vi "OLD_Dashboard_Main_Fixed_1280_768.vi"() -> ()   [LabVIEW 2025]
uses:
  frobotics-2025RobotCode/2025ReefBot/Intake/IntakeStates.ctl
  frobotics-2025RobotCode/2025ReefBot/NewAuto/NewAutoStepTypeEnum.ctl
  <vilib>/event_ctls.llb/eventvkey.ctl
  frobotics-2025RobotCode/Dashboard-Testing/Dash_Globals.vi
  <vilib>/Rock Robotics/Network Tables/NT Read Boolean.vi
  <vilib>/Rock Robotics/Network Tables/NT Write Boolean.vi
  <vilib>/Rock Robotics/WPI/Dashboard/WPI_DashboardLogging Global.vi
  <vilib>/Rock Robotics/WPI/ThirdParty/JAS_Junk/TrajLib/Trajectory_Library.lvlib
panel:
  in  "Camera Settings Right":T1={"Frame Rate"=30, "Compression"=30, "Size"=1, "DB Camera Config"=FALSE} {"Frame Rate" scale=1.0..30.0; "Compression" scale=100.0..-1.0; "Size" items=["640x480", "320x240", "160x120"]}
  in  "Camera Name Right":string(combo)="No Camera Selection"
  out "Camera Perf":string
  in  "Camera Settings":T1={"Frame Rate"=30, "Compression"=30, "Size"=1, "DB Camera Config"=FALSE} {"Frame Rate" scale=1.0..30.0; "Compression" scale=100.0..-1.0; "Size" items=["640x480", "320x240", "160x120"]}
  in  "TCP":refnum<k5>
  in  "Rec Mode":enum32{"Stop", "Record", "Playback"}(radio)
  out "Robot IP":string
  out "Image Message":string="Timeout in Camera Communications"
  in  "Dashboard Tab":T2(tab)
  out "Human Fast Turn":bool
  out "H Traj Orient Deg":dbl format="%11.2f"
  out "H Traj Y Ft":dbl format="%11.2f"
  out "H Traj X Ft":dbl format="%11.2f"
  out "Human Slow Mode":bool
  out "Human Field Orient":bool
  out "A String":string
  out "P3":dbl format="%11.2f"
  out "Function":T3
  out "A Step":i64 format="%11.0f"
  out "P2":dbl format="%11.2f"
  out "P1":dbl format="%11.2f"
  out "TO":dbl format="%11.2f"
  out "Vision Targets Found":bool
  out "Climb Position":dbl format="%15.2f"
  out "Climb Status":string
  out "Fully Pulled":bool
  out "Fully Reached":bool
  out "Intake State":T4
  out "Have Algae":bool
  out "Have Coral":bool
  out "W PV":dbl(slide) scale=-90.0..90.0
  out "W SP":dbl(slide) scale=-90.0..90.0
  out "W Hi Clamp":bool
  out "W Lo Clamp":bool
  out "W On Tgt":bool
  out "W Motor":dbl format="%11.2f"
  out "W Pos Deg":dbl format="%12.1f"
  out "W Dmd Deg":dbl format="%12.1f"
  out "I PV":dbl(slide) scale=0.0..26.0
  out "I SP":dbl(slide) scale=0.0..26.0
  out "I Lo Clamp":bool
  out "I Lo Lim":bool
  out "I Hi Lim":bool
  out "I On Tgt":bool
  out "I Motor":dbl format="%11.2f"
  out "I Pos In":dbl format="%12.1f"
  out "I Dmd In":dbl format="%12.1f"
  in  "Select Auto":string(combo)="Select Autonomous ..."
  out "NT Connection":bool
  out "Mode":T5(ring)=enum."Auto Disabled"
  out "Right Camera Perf":cluster{"Bandwidth (Mbps)":dbl, "FPS":dbl}
  out "Selected Auto":string
  out "O PV":dbl(slide) scale=0.0..52.0
  out "O SP":dbl(slide) scale=0.0..52.0
  out "O Lo Lim":bool
  out "O Hi Lim":bool
  out "O On Tgt":bool
  out "O Motor":dbl format="%11.2f"
  out "O Pos In":dbl format="%12.1f"
  out "O Dmd In":dbl format="%12.1f"
  out "Camera Image Right":T6(plugin-control)
  out "AlgSensOffDlyFB":dbl
  in  "AlgSensOffDly":dbl
  out "AlgSensOnDlyFB":dbl
  in  "AlgSensOnDly":dbl
  out "AlgHoldMtrFB":dbl
  in  "AlgHoldMtr":dbl
  in  "Alg Update":bool
  out "AlgIntakeMtrFB":dbl
  in  "AlgIntakeMtr":dbl
  out "Max Amb FB":dbl
  in  "Max Amb":dbl
  out "I Orient Deg FB":dbl
  in  "Init Orient Deg":dbl
  out "InitYPosFt FB":dbl
  in  "InitYPos Ft":dbl
  in  "Vision Update":bool
  out "InitXPos Ft FB":dbl
  in  "InitXPos Ft":dbl
  out "RL Enable FB":bool
  in  "RL Enable":bool
  out "Y Acc M/S2 FB":dbl
  in  "Y Acc M/S2":dbl
  in  "RL Update":bool
  out "X Acc M/S2 FB":dbl
  in  "X Acc M/S2":dbl
  in  "RA Update":bool
  out "R Starting Angle FB":dbl
  in  "R Starting Angle":dbl
  in  "LQR":bool
  in  "Filter":bool
  out "Wrist Chart":T7(graph)
  out "Kp Calc":dbl
  out "Kg FB":dbl
  in  "Kg":dbl
  out "Kd FB":dbl format="%#_7g"
  in  "Kd":dbl format="%#_7g"
  out "Output Max FB":dbl
  in  "Output Max":dbl
  out "Output DB FB":dbl
  in  "Output DB":dbl
  out "Error DB FB":dbl
  in  "Error DB":dbl
  in  "WR Tune Update":bool
  out "Error Thres FB":dbl
  in  "Error Thres":dbl
  out "Filt FB":bool
  out "LQR FB":bool
  in  "Test Slider":dbl(slide) scale=0.0..100.0 scale format="%#_3g"
  in  "On/Off":bool caption="Solenoid"
  in  "Test Name":u16(ring) items=["Select the test to run..."]
  in  "Test Tree":string(tree)
  in  "Motor":cluster{"Value":dbl, "Enable":bool} {"Value" scale=-1.0..1.0 scale format="%#_3g"}
  out "Progress":T8 {"Test Progress" scale=0.0..100.0}
  in  "Rev/Fwd":cluster{"Forward":bool, "Reverse":bool}
  in  "Test Ring":u16(ring) items=["Monochrome", "Color"]
  in  "CheckList":i32(listbox)
  out "Tree":string(tree)
  out "Camera Image":T6(plugin-control)
  out "Background":bool
  in  "Camera Name":string(combo)="No Camera Selection"
  # "HW"
  # "HW"
  # "Human"
  # "Auto"
  # "VISION"
  # "CLIMB"
  # "INTAKE"
  # "WRIST"
  # "INNER ELEV"
  # "OUTER ELEV"
  # "Intake Algae Tuning"
  # "Vision Tuning"
  # "Drive Rate Limiting"
  # "Initial Robot Angle"
  # "Wrist Tuning"
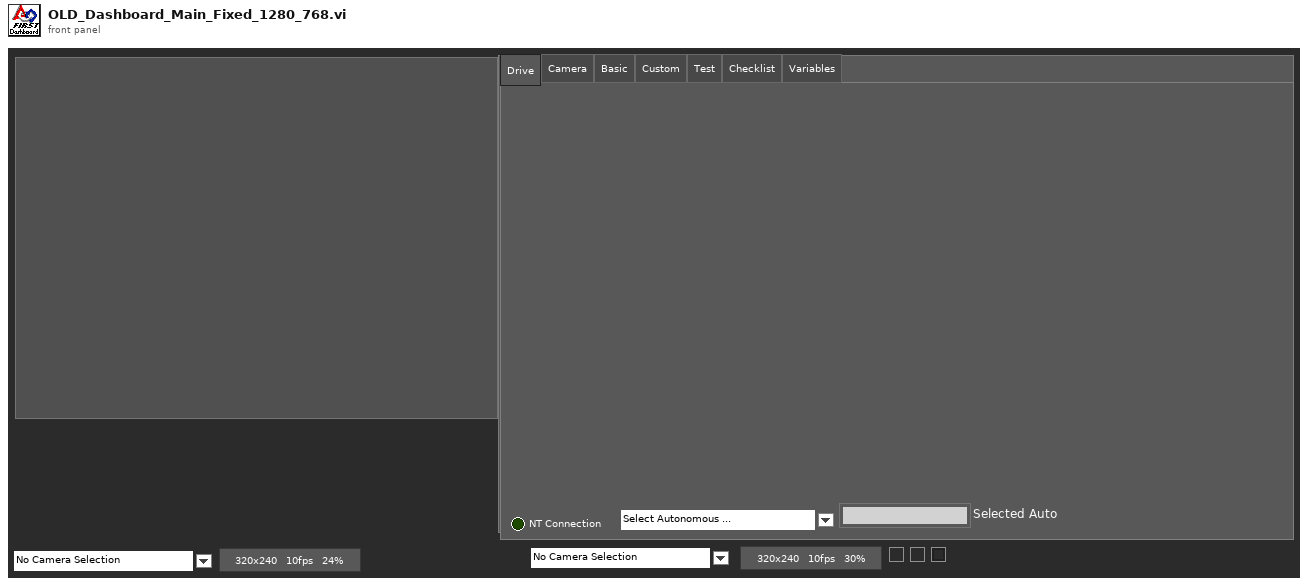
[diagram p1: front panel]
types:
  T1 = cluster{"Frame Rate":i32, "Compression":i32, "Size":u16, "DB Camera Config":bool}
  T2 = enum32{"Drive", "Camera", "Basic", "Custom", "Test", "Checklist", "Variables"}
  T3 = typedef "NewAutoStepTypeEnum.ctl" = enum16{"DriveStraight", "DriveTurn", "FollowAbsoluteTrajectory", "FollowRelativeTrajectory", "AutoWait", "ElevToRest", "ElevToFloor", "ElevToSource", "ElevToL1", "ElevToL2", "ElevToL3", "ElevToL4", "ElevToAlgae1", "ElevToAlgae2", "ElevToBarge", "ElevCancel", "IntakeCoral", "IntakeAlgae", "IntakeDepositCoral", "IntakeDepositAlgae", "IntakeCancel", "ElevRestWait", "ElevFloorWait", "ElevSourceWait", "ElevL1Wait", "ElevL2Wait", "ElevAlgae1Wait", "ElevL3Wait", "ElevAlgae2Wait", "ElevL4Wait", "ElevBargeWait", "IntakeWait", "FollowAbsTrajWithTimedCmd", "FollowRelTrajWithTimedCmd"}
  T4 = typedef "IntakeStates.ctl" = enum16{"Start", "WaitForCommand", "IntakeCoral", "IntakeAlgae", "WaitForCoral", "WaitForAlgae", "DepositCoral", "DepositAlgae", "DepositCoralTimer", "DepositAlgaeTimer"}
  T5 = enum8{"Tele-Op Disabled", "Tele-Op Enabled", "Auto Disabled", "Auto Enabled", "Test Disabled", "Test Enabled", "Disconnected", "No Code", "E-Stop"}
  T6 = typedef "IMAQ Image.ctl" = refnum<image>
  T7 = cluster{"WristSetpointDeg":dbl, "WristPosDeg":dbl, "WristMotorDmd":dbl, "WristGravityCompMotorDmd":dbl}
  T8 = cluster{"Test Progress":u8, "Test Progress Text":string}
  T9 = cluster{"Save Path":path, "Interval (s)":dbl, "Keep":i32}
  T10 = typedef "Image Type" = u32
  T11 = enum32{"Drive", "Camera", "Basic", "Custom", "Test", "Commands", "Checklist", "Variables"}
  T12 = cluster{"Error Strings":string, "Disable Counts":cluster{u16, u16}, "Rail Faults":cluster{u16, u16, u16}, "Robot IP":string, "DB Mode":u8, "Event Info":cluster{"Name":string, "Type":u8, "Number":u16, "Replay":u8}}
  T13 = cluster{"Storage":cluster{"Disk Free":u64, "RAM Block":u32, "RAM free":u32}, "CPU Utilization":cluster{"CPU % ISR":sgl, "CPU % Time Crit":sgl, "CPU % Timed Str":sgl, "CPU % High":sgl, "CPU % Above":sgl, "CPU % Normal":sgl, "CPU % Low":sgl}, "CAN":cluster{"% Bus Utilization":sgl, "Bus Off Cnt":u32, "TX_FIFO Full Cnt":u32, "Receive Error Cnt":u8, "Transmit Error Cnt":u8}, "HID":cluster{"HID Outputs":u32, "Rumble Low":u16, "Rumble High":u16}[]}
  T14 = cluster{"Status bits":cluster{"Test Mode":bool, "Autonomous":bool, "Enabled":bool, "Code Start":bool, "Brownout":bool, "Reserved 2":bool, "Reserved 3":bool, "E-Stop":bool}, "Code Trace":cluster{"Disabled":bool, "TeleOp":bool, "Auto":bool, "Test":bool}, "Controller Type":enum16{"unknown", "cRIO", "roboRio"}, "Code?":enum16{"unknown", "noCode", "code"}, "Battery V":dbl}
  T15 = cluster{"Control Bits":cluster{"TestMode":bool, "Autonomous":bool, "Enabled":bool, "FMS Present":bool, bool, bool, bool, "E-Stop":bool}, "Team Station ":u8, "Countdown":sgl, "Joystick Values":cluster{"Axes":dbl[], "Buttons":bool[], "POVs":i16[]}[]}
  T16 = cluster{"Camera Image":refnum<vi>, "Dashboard Tab":refnum<vi>, "Background":refnum<vi>, "Rec Mode":refnum<vi>, "Test Slider":refnum<vi>, "On/Off ":refnum<vi>, "Test Ring":refnum<vi>, "Rev/Fwd":refnum<vi>, "Test Name":refnum<vi>, "Motor":refnum<vi>, "Progress":refnum<vi>, "CheckList":refnum<vi>, "Tree":refnum<vi>, "Test Tree":refnum<vi>, "Camera Settings":refnum<vi>, "Camera Name":refnum<vi>, "Camera Perf":refnum<vi>, "Camera Settings Right":refnum<vi>, "Camera Name Right":refnum<vi>, "Camera Image Right":refnum<vi>}
  T17 = cluster{"Global Rectangle":i32[], "Contours":cluster{"Contour Type":u32, "ROI Type":u32, "Points":i32[]}[]}
  T18 = cluster{"Camera Name":string, string, "Saved DB Images Info":cluster{"Save Path":path, "Interval (s)":dbl, "Keep":i32}}
  T19 = cluster{"Camera Name Right":string, string, "Saved DB Images Info":cluster{"Save Path":path, "Interval (s)":dbl, "Keep":i32}}
  T20 = cluster{"Operation":enum16{"Update", "Clear"}, "Color Box":u32}[]
  T21 = typedef "eventvkey.ctl" = enum16{"ASCII", "Enter", "Return", "Shift", "Ctrl", "Alt", "Cmd", "Opt", "Caps", "NumLock", "Clear", "Break", "Up", "Down", "Left", "Right", "Insert", "Delete", "Home", "End", "PageUp", "PageDown", "Escape", "Help", "Pause", "ScrollLock", "F1", "F2", "F3", "F4", "F5", "F6", "F7", "F8", "F9", "F10", "F11", "F12", "F13", "F14", "F15", "F16", "F17", "F18", "F19", "F20", "F21", "F22", "F23", "F24", "Play", "VolumeUp", "VolumeDown", "Mute", "Two Byte Char"}
  T22 = cluster{"Image Size":bool, "Image Type":bool, "Pixel Value":bool, "ROI Information":bool, "Zoom Factor":bool}
  T23 = cluster{"Operation":enum16{"Update", "Clear"}, "Color Box":u32}
  T24 = cluster{"Shift":bool, "Ctrl":bool, "Alt":bool, "Cmd":bool, "Opt":bool}
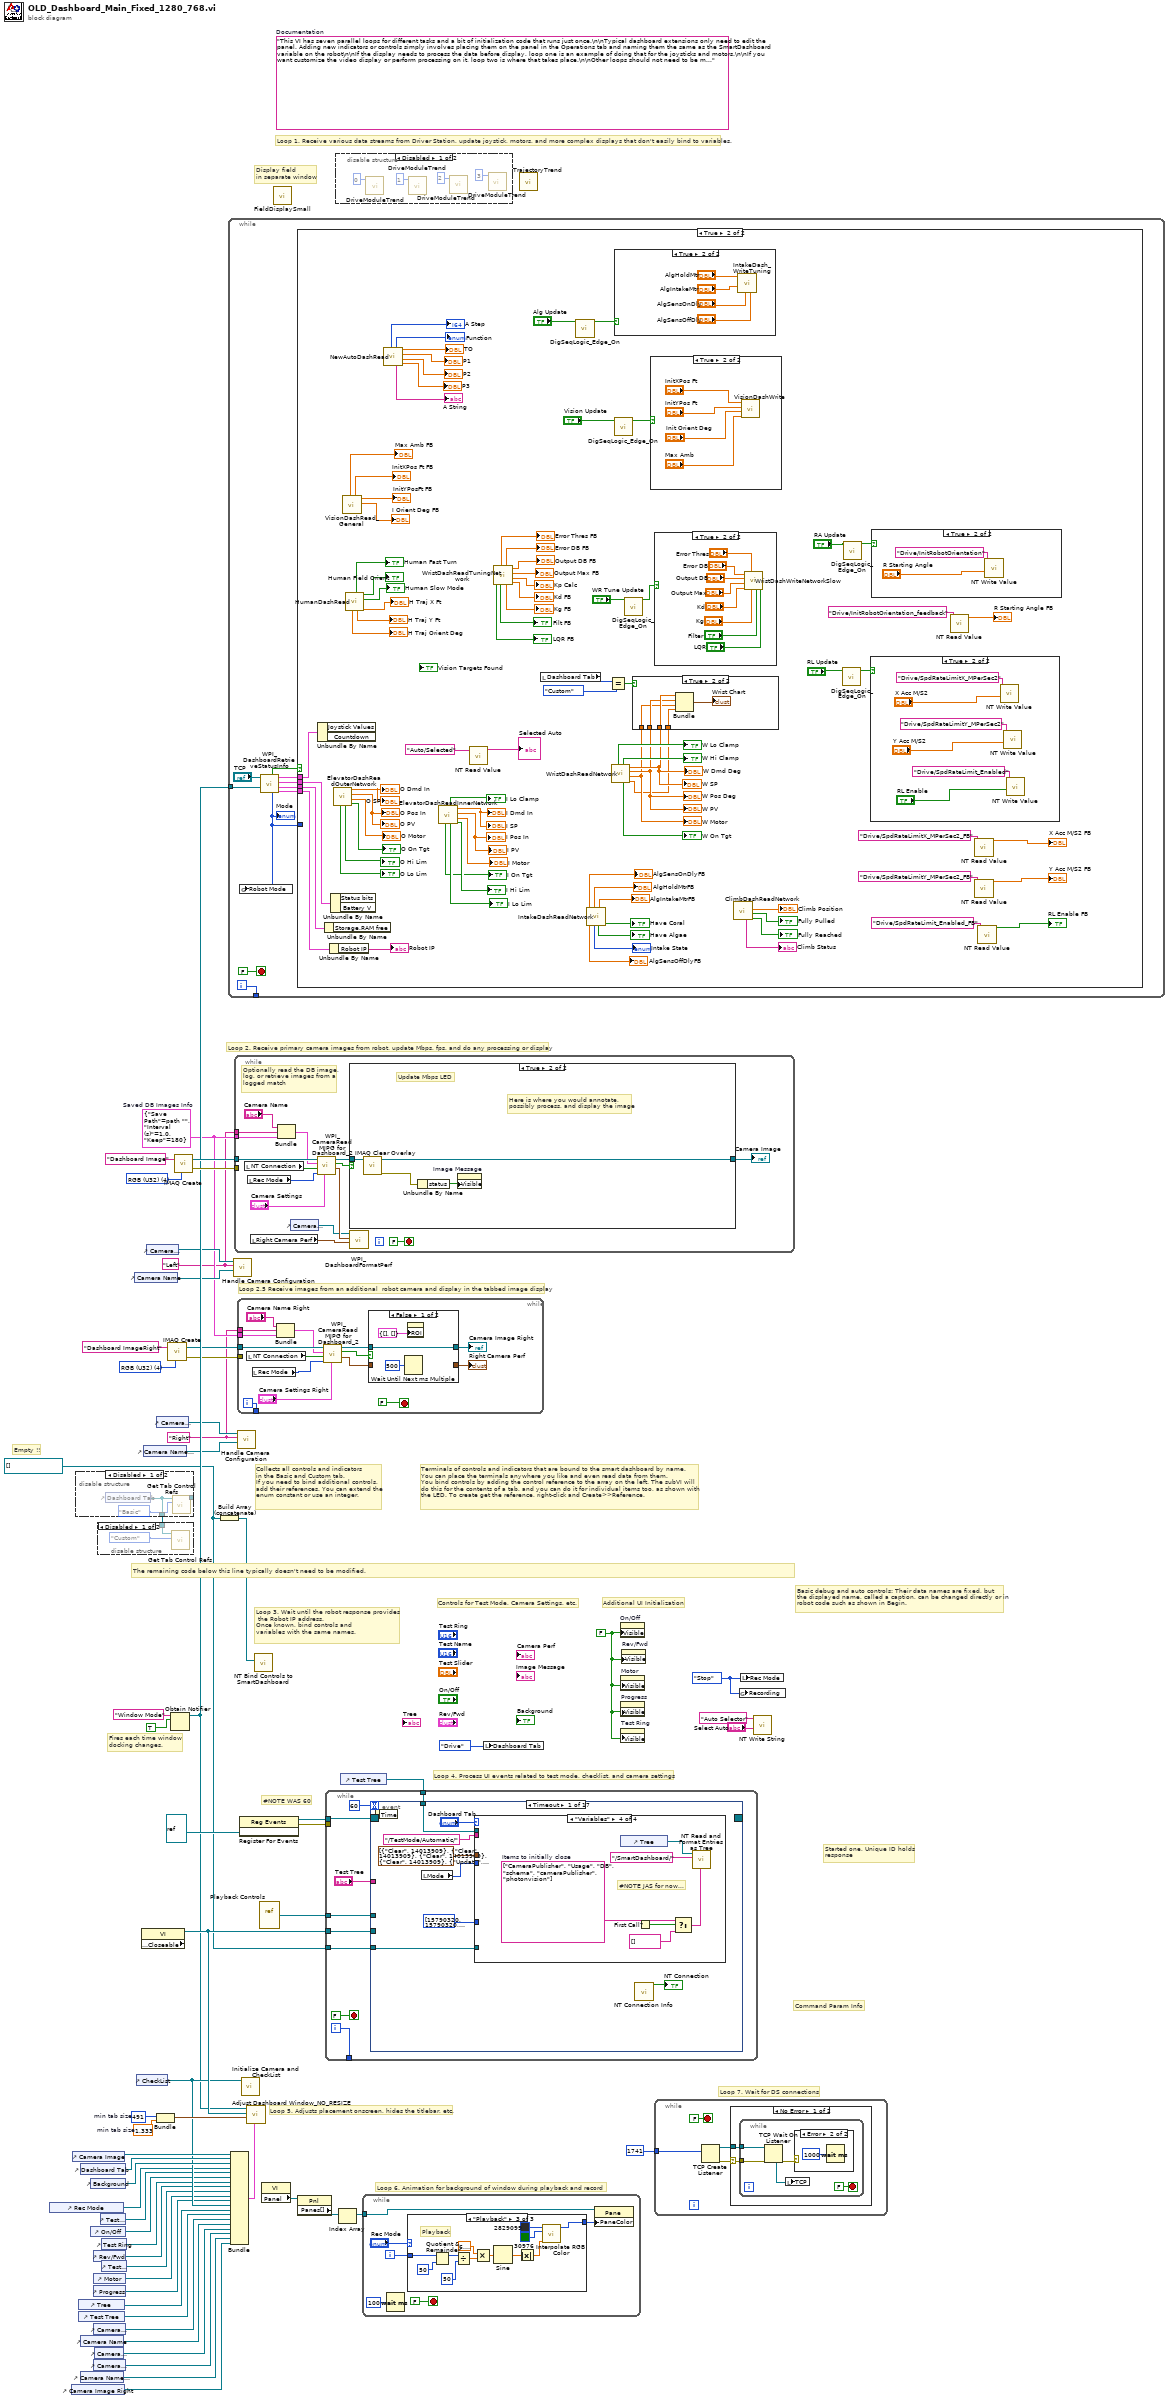
[diagram p0: block diagram]
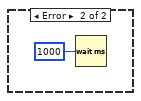
[diagram p7: hidden frame]
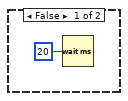
[diagram p8: hidden frame]
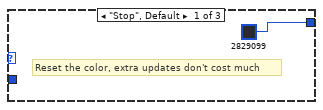
[diagram p15: hidden frame]
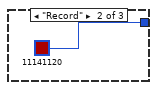
[diagram p16: hidden frame]
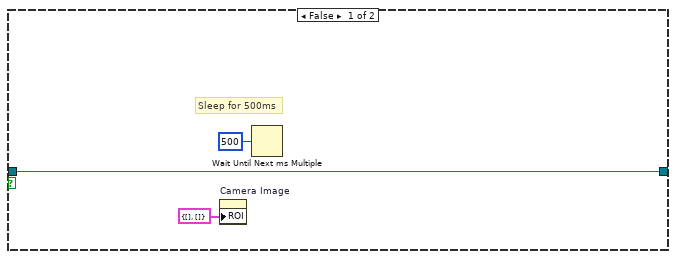
[diagram p17: hidden frame]
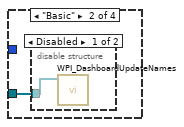
[diagram p19: hidden frame]
diagram:
  w1 = refnum<vi>[] [] ("ControlsOnPage")
  w4 = T9 {"Save Path"=path "", "Interval (s)"=1.0, "Keep"=180}  # Saved DB Images Info
  w3 = "Right"
  w2 = "Left"
  w12 = T10 4 items=["Grayscale (U8)", "Grayscale (I16)", "Grayscale (SGL)", "Complex (CSG)", "RGB (U32)", "HSL (U32)", "RGB (U64)"] ("Image Type")
  w40 = 491  # min tab size
  w39 = 1.333  # min tab size
  w46 = enum32{"Stop", "Record", "Playback"}."Stop" ("Rec Mode")
  w24 = FALSE ("Visible")
  (unwired) "This VI has seven parallel loops for different tasks and a bit of initialization code that runs just once.\n\nTypical dashboard extensions only need to edit the panel. Adding new indicators or controls simply involves placing them on the panel in the Operations tab and naming them the same as the SmartDashboard variable on the robot\n\nIf the display needs to process the data before display, loop one is an example of doing that for the joysticks and motors.\n\nIf you want customize the video display or perform processing on it, loop two is where that takes place.\n\nOther loops should not need to be modified. They are pretty standard, and document the task they perform."  # Documentation
  w60 = T10 4 items=["Grayscale (U8)", "Grayscale (I16)", "Grayscale (SGL)", "Complex (CSG)", "RGB (U32)", "HSL (U32)", "RGB (U64)"] ("Image Type")
  # "#NOTE WAS 60"
  # "Empty !!"
  # "Display field\nin separate window"
  # "Loop 2.5 Receive images from an additional  robot camera and display in the tabbed image display"
  # "Command Param Info"
  # "Started one, Unique ID holds\nresponse"
  # "Loop 7. Wait for DS connections"
  # "Basic debug and auto controls: Their data names are fixed, but\nthe displayed name, called a caption, can be changed directly or in\nrobot code such as shown in Begin."
  # "Controls for Test Mode, Camera Settings, etc."
  # "Additional UI Initialization"
  # "Loop 6. Animation for background of window during playback and record"
  # "Fires each time window\ndocking changes."
  # "Collects all controls and indicators\nin the Basic and Custom tab.\nIf you need to bind additional controls,\nadd their references. You can extend the\nenum constant or use an integer."
  # "The remaining code below this line typically doesn't need to be modified."
  # "Loop 4. Process UI events related to test mode, checklist, and camera settings"
  # "Terminals of controls and indicators that are bound to the smart dashboard by name.\nYou can place the terminals anywhere you like and even read data from them.\nYou bind controls by adding the control reference to the array on the left. The subVI will\ndo this for the contents of a tab, and you can do it for individual items too, as shown with\nthe LED. To create get the reference, right-click and Create>>Reference."
  # "Loop 3. Wait until the robot response provides\n the Robot IP address.\nOnce known, bind controls and\nvariables with the same names."
  # "Loop 5. Adjusts placement onscreen, hides the titlebar, etc."
  # "Loop 1. Receive various data streams from Driver Station, update joystick, motors, and more complex displays that don't easily bind to variables."
  # "Loop 2. Receive primary camera images from robot, update Mbps, fps, and do any processing or display"
  n1 = control-ref of="Rec Mode"() -> (w30:refnum<vi>)
  n2 = control-ref of="Camera Image Right"() -> (w5:refnum<vi>)
  n3 = control-ref of="Camera Image"() -> (w42:refnum<vi>)
  n4 = disable-structure shown="Disabled" {
    disable-tunnel: [w63 _] -> w44
    disable-tunnel: [w62 _] -> _
    frame Disabled {
      n5 = control-ref of="Dashboard Tab"() -> (w63:refnum<vi>)
      n6 = call <vilib>:"Get Tab Control Refs.vi"("Page Index"=T11."Basic" ("Dashboard Tab"), "TabControl in"=w63) -> ("ControlsOnPage"=w62:refnum<vi>[])  [unwired: 9 in]
    }
    frame Enabled {
    }
  }
  n7 = control-ref of="Tree"() -> (w34:refnum<vi>)
  n8 = control-ref of="Test Tree"() -> (w33:refnum<vi>)
  n9 = control-ref of="Dashboard Tab"() -> (w41:refnum<vi>)
  n10 = control-ref of="Camera Name"() -> (w17:refnum<vi>)
  n11 = control-ref of="Camera Name Right"() -> (w6:refnum<vi>)
  n12 = control-ref of="Background"() -> (w37:refnum<vi>)
  n13 = control-ref of="On/Off"() -> (w28:refnum<vi>)
  n14 = control-ref of="Progress"() -> (w25:refnum<vi>)
  n15 = control-ref of="Camera Settings"() -> (w18:refnum<vi>)
  n16 = control-ref of="Camera Settings Right"() -> (w7:refnum<vi>)
  n17 = control-ref of="Rev/Fwd"() -> (w26:refnum<vi>)
  n18 = control-ref of="Motor"() -> (w31:refnum<vi>)
  n19 = control-ref of="Camera Perf"() -> (w16:refnum<vi>)
  n20 = disable-structure shown="Disabled" {
    disable-tunnel: w44 -> [w65 _]
    frame Disabled {
      n21 = call <vilib>:"Get Tab Control Refs.vi"("Page Index"=T11."Custom" ("Dashboard Tab"), "TabControl in"=w65) -> ()  [unwired: 9 in, 1 out]
    }
    frame Enabled {
    }
  }
  n22 = control-ref of="Test Slider"() -> (w29:refnum<vi>)
  n23 = control-ref of="Test Ring"() -> (w27:refnum<vi>)
  n24 = control-ref of="Test Name"() -> (w32:refnum<vi>)
  n25 = control-ref of="Camera Name"() -> (w19:refnum<vi>)
  n26 = control-ref of="CheckList"() -> (w35:refnum<vi>)
  n27 = property class="VI" props=["Front Panel.Closeable"]() -> (reference out=w45:refnum<vi>)  [unwired: 2 in, 2 out]
  n28 = control-ref of="Camera Name Right"() -> (w8:refnum<vi>)
  n29 = control-ref of="Camera Settings"() -> (w20:refnum<vi>)
  n30 = control-ref of="Camera Settings Right"() -> (w9:refnum<vi>)
  n31 = Bundle("min tab size"=w40, "min tab size"=w39) -> (w38:cluster{"min tab size":i32, "min tab size":dbl})  [unwired: 1 in]
  n32 = call "IMAQ Create"("Image Name"="Dashboard ImageRight", "Image Type"=w12) -> ("New Image"=w11:T6, "error out"=w10:errorcluster)  [unwired: 2 in, 1 out]
  n33 = Obtain Notifier(name (unnamed)="Window Mode", notification data type=TRUE) -> (notifier out=w23:refnum<notifier>)  [unwired: 2 in, 2 out]
  n34 = call "IMAQ Create"("Image Name"="Dashboard Image", "Image Type"=w60) -> ("New Image"=w58:T6, "error out"=w57:errorcluster)  [unwired: 2 in, 1 out]
  n35 = Build Array (concatenate)(w1) -> (w43:refnum<vi>[])
  n36 = while {
    tunnel: [w74] -> _
    tunnel: w23 -> [w67]
    i -> [w74]
    stop <- FALSE stop-if-true
    n37 = call <vilib>:"WPI_DashboardRetrieveStatusInfo.vi"("Window Mode Notifier"=w67, "TCP Cnx"="TCP") -> ("Power and Errors"=w69:T12, "Robot Metrics"=w72:T13, "Status Info"=w73:T14, "Control Info"=w70:T15, "Robot Mode"=w66:T5, "Process?"=w71:bool)  [unwired: 4 in]
    "Mode" <- w66
    n38 = global write "Dash_Globals.vi" "Robot Mode"(w66) -> ()
    n39 = case shown="True" w71 {
      tunnel: w73 -> [_ w161]
      tunnel: w72 -> [_ w160]
      tunnel: w70 -> [_ w159]
      tunnel: w69 -> [_ w158]
      tunnel: w66 -> [_ _]
      frame False {
        n40 = Wait (ms)(milliseconds to wait=u32 20) -> ()  [unwired: 1 out]
      }
      frame True {
        n41 = Unbundle By Name(w159) -> ()  [unwired: 2 out]
        n42 = Unbundle By Name(w160) -> ()  [unwired: 1 out]
        n43 = Unbundle By Name(w158) -> ("Robot IP"=→"Robot IP":string)
        n44 = Unbundle By Name(w161) -> ()  [unwired: 2 out]
        n45 = call "ElevatorDashReadOuterNetwork.vi"() -> ("OuterOnTarget"=→"O On Tgt":bool, "OuterMotorOutput"=→"O Motor":dbl, "OuterPositionHeight"=→"O PV" →"O Pos In":dbl, "OuterPosDemandHeight"=→"O SP" →"O Dmd In":dbl, "OuterHighLimitSwitch"=→"O Hi Lim":bool, "OuterLowLimitSwitch"=→"O Lo Lim":bool)  [unwired: 6 in]
        n46 = call "VisionDashRead_General.vi"() -> ("InitOrientDeg"=→"I Orient Deg FB":dbl, "InitYFt"=→"InitYPosFt FB":dbl, "InitXFt"=→"InitXPos Ft FB":dbl, "MaxAmbiguity"=→"Max Amb FB":dbl)  [unwired: 4 in, 4 out]
        n47 = call "HumanDashRead.vi"() -> ("TrajDestX_Ft"=→"H Traj X Ft":dbl, "SlowMode"=→"Human Slow Mode":bool, "FieldOriented"=→"Human Field Orient":bool, "TrajDestY_Ft"=→"H Traj Y Ft":dbl, "FastMode"=→"Human Fast Turn":bool, "TrajDestAng_Deg"=→"H Traj Orient Deg":dbl)  [unwired: 5 in, 1 out]
        n48 = call "NewAutoDashRead.vi"() -> ("P3"=→"P3":dbl, "P2"=→"P2":dbl, "P1"=→"P1":dbl, "Timeout"=→"TO":dbl, "StepString"=→"A String":string, "StepType"=→"Function":T3, "StepIndex"=→"A Step":i64)  [unwired: 5 in]
        n49 = call "ElevatorDashReadInnerNetwork.vi"() -> ("Stage3HighLimitSwitch"=→"I Hi Lim":bool, "Stage3MotorOutput"=→"I Motor":dbl, "Stage3PositionHeight"=→"I Pos In" →"I PV":dbl, "Stage3PosDemandHeight"=→"I Dmd In" →"I SP":dbl, "Stage3LowLimitSwitch"=→"I Lo Lim":bool, "Stage3LowWristClampActive"=→"I Lo Clamp":bool, "Stage3OnTarget"=→"I On Tgt":bool)  [unwired: 5 in]
        n50 = call-poly <vilib>:"NT Read Value.vi"("name"="Auto/Selected") -> ("value"=→"Selected Auto":string)  [unwired: 8 in, 2 out]
        n51 = call "WristDashReadTuningNetwork.vi"() -> ("Tune_Kd"=→"Kd FB":dbl, "Tune_Kp"=→"Kp Calc":dbl, "Tune_OutMax"=→"Output Max FB":dbl, "Tune_OutDb"=→"Output DB FB":dbl, "Tune_Kg"=→"Kg FB":dbl, "Tune_ErrDb"=→"Error DB FB":dbl, "FilterDerivative"=→"Filt FB":bool, "Tune_ErrThres"=→"Error Thres FB":dbl, "UseLQR"=→"LQR FB":bool)  [unwired: 3 in]
        n52 = local read "Dashboard Tab"() -> (w109:T2)
        n53 = call <vilib>:"DigSeqLogic_Edge_On.vi"("Input"="Alg Update") -> ("On Edge"=w82:bool)  [unwired: 10 in]
        n54 = call "IntakeDashReadNetwork.vi"() -> ("HaveCoralSensor"=→"Have Coral":bool, "HaveAlgaeSensor"=→"Have Algae":bool, "AlgaeIntakeMtr"=→"AlgIntakeMtrFB":dbl, "CurrentState"=→"Intake State":T4, "AlgaeHoldMtr"=→"AlgHoldMtrFB":dbl, "AlgaeSensorOffDelaySec"=→"AlgSensOffDlyFB":dbl, "AlgaeSensorOnDelaySec"=→"AlgSensOnDlyFB":dbl)  [unwired: 2 in, 3 out]
        n55 = Equal?(x=w109, y=T2."Custom") -> (x = y?=w110:bool)
        n56 = call "WristDashReadNetwork.vi"() -> ("WristGravityCompMotorDmd"=w102:dbl, "WristMotorDmd"=w105:dbl, "WristPosDeg"=w106:dbl, "WristSetpointDeg"=w107:dbl, "WristAtSetpoint"=→"W On Tgt":bool, "WristProtectHighClampActive"=→"W Hi Clamp":bool, "WristProtectLowClampActive"=→"W Lo Clamp":bool)  [unwired: 5 in]
        "W Dmd Deg" <- w107
        "W Pos Deg" <- w106
        "W Motor" <- w105
        "W SP" <- w107
        "W PV" <- w106
        n57 = case shown="True" w82 {
          frame False {
          }
          frame True {
            n58 = call "IntakeDash_WriteTuning.vi"("AlgaeSensorOffDelaySec"="AlgSensOffDly", "AlgaeSensorOnDelaySec"="AlgSensOnDly", "AlgaeIntakeMtr"="AlgIntakeMtr", "AlgaeHoldMtr"="AlgHoldMtr") -> ()  [unwired: 8 in]
          }
        }
        n59 = call <vilib>:"DigSeqLogic_Edge_On.vi"("Input"="Vision Update") -> ("On Edge"=w100:bool)  [unwired: 10 in]
        n60 = call <vilib>:"DigSeqLogic_Edge_On.vi"("Input"="WR Tune Update") -> ("On Edge"=w112:bool)  [unwired: 10 in]
        n61 = case shown="True" w110 {
          tunnel: w107 -> [_ w173]
          tunnel: w106 -> [_ w172]
          tunnel: w105 -> [_ w171]
          tunnel: w102 -> [_ w170]
          frame False {
          }
          frame True {
            n62 = Bundle("WristSetpointDeg"=w173, "WristPosDeg"=w172, "WristMotorDmd"=w171, "WristGravityCompMotorDmd"=w170) -> (→"Wrist Chart":T7)  [unwired: 1 in]
          }
        }
        n63 = case shown="True" w100 {
          frame False {
          }
          frame True {
            n64 = call "VisionDashWrite.vi"("MaxAmbiguity"="Max Amb", "InitialOrientationDeg"="Init Orient Deg", "InitialYPositionFt"="InitYPos Ft", "InitialXPositionFt"="InitXPos Ft") -> ()  [unwired: 8 in]
          }
        }
        n65 = case shown="True" w112 {
          frame False {
          }
          frame True {
            n66 = call "WristDashWriteNetworkSlow.vi"("UseLQR"="LQR", "FilterDerivative"="Filter", "Tune_Kg"="Kg", "Tune_ErrThres"="Error Thres", "Tune_Kd"="Kd", "Tune_OutMax"="Output Max", "Tune_OutDb"="Output DB", "Tune_ErrDb"="Error DB") -> ()  [unwired: 4 in]
          }
        }
        n67 = call "ClimbDashReadNetwork.vi"() -> ("ReachLimit"=→"Fully Reached":bool, "PullLimit"=→"Fully Pulled":bool, "SensorPosition"=→"Climb Position":dbl, "ClimbStatus"=→"Climb Status":string)  [unwired: 7 in, 1 out]
        n68 = call <vilib>:"DigSeqLogic_Edge_On.vi"("Input"="RL Update") -> ("On Edge"=w126:bool)  [unwired: 10 in]
        n69 = call <vilib>:"DigSeqLogic_Edge_On.vi"("Input"="RA Update") -> ("On Edge"=w128:bool)  [unwired: 10 in]
        n70 = case shown="True" w126 {
          frame False {
          }
          frame True {
            n71 = call-poly <vilib>:"NT Write Value.vi"("value"="X Acc M/S2", "name"="Drive/SpdRateLimitX_MPerSec2") -> ()  [unwired: 9 in, 1 out]
            n72 = call-poly <vilib>:"NT Write Value.vi"("value"="Y Acc M/S2", "name"="Drive/SpdRateLimitY_MPerSec2") -> ()  [unwired: 9 in, 1 out]
            n73 = call-poly <vilib>:"NT Write Value.vi"("value"="RL Enable", "name"="Drive/SpdRateLimit_Enabled") -> ()  [unwired: 9 in, 1 out]
          }
        }
        n74 = case shown="True" w128 {
          frame False {
          }
          frame True {
            n75 = call-poly <vilib>:"NT Write Value.vi"("value"="R Starting Angle", "name"="Drive/InitRobotOrientation") -> ()  [unwired: 9 in, 1 out]
          }
        }
        n76 = call-poly <vilib>:"NT Read Value.vi"("name"="Drive/InitRobotOrientation_feedback") -> ("value"=→"R Starting Angle FB":dbl)  [unwired: 8 in, 2 out]
        n77 = call-poly <vilib>:"NT Read Value.vi"("name"="Drive/SpdRateLimitX_MPerSec2_FB") -> ("value"=→"X Acc M/S2 FB":dbl)  [unwired: 8 in, 2 out]
        n78 = call-poly <vilib>:"NT Read Value.vi"("name"="Drive/SpdRateLimitY_MPerSec2_FB") -> ("value"=→"Y Acc M/S2 FB":dbl)  [unwired: 8 in, 2 out]
        n79 = call-poly <vilib>:"NT Read Value.vi"("name"="Drive/SpdRateLimit_Enabled_FB") -> ("value"=→"RL Enable FB":bool)  [unwired: 8 in, 2 out]
      }
    }
  }
  n80 = Bundle("Camera Image"=w42, "Dashboard Tab"=w41, "Background"=w37, "Rec Mode"=w30, "Test Slider"=w29, "On/Off"=w28, "Test Ring"=w27, "Rev/Fwd"=w26, "Test Name"=w32, "Motor"=w31, "Progress"=w25, "CheckList"=w35, "Tree"=w34, "Test Tree"=w33, "Camera Settings"=w18, "Camera Name"=w17, "Camera Perf"=w16, "Camera Settings Right"=w7, "Camera Name Right"=w6, "Camera Image Right"=w5) -> (w36:T16)  [unwired: 1 in]
  n81 = call "Handle Camera Configuration.vi"("CameraNameRef"=w19, "Display Name"=w2, "ClusterRef"=w20) -> ()  [unwired: 9 in]
  n82 = while {
    tunnel: w58 -> [w204]
    tunnel: w57 -> [_]
    tunnel: w4 -> [w197]
    tunnel: w2 -> [w194]
    stop <- FALSE stop-if-true
    # "Optionally read the DB image,\nlog, or retrieve images from a\nlogged match"
    n83 = local read "NT Connection"() -> (w198:bool)
    n84 = local read "Rec Mode"() -> (w201:enum32{"Stop", "Record", "Playback"})
    n85 = local read "Right Camera Perf"() -> (w192:cluster{"Bandwidth (Mbps)":dbl, "FPS":dbl})
    n86 = Bundle("Camera Name"="Camera Name", w194, "Saved DB Images Info"=w197) -> (w196:T18)  [unwired: 1 in]
    n87 = control-ref of="Camera Perf"() -> (w191:refnum<vi>)
    n88 = call <vilib>:"WPI_CameraRead MJPG for Dashboard_2.vi"("Camera Settings"="Camera Settings", "Rec Mode"=w201, "NT Connection"=w198, "Capture Info"=w196, "Image in"=w204) -> ("perf info"=w193:cluster{"Bandwidth (Mbps)":dbl, "fps":dbl}, "Active"=w202:bool, "Image\\ out"=w203:T6)  [unwired: 4 in]
    n89 = case shown="True" w202 {
      tunnel: w203 -> [w207 w210]
      tunnel: [w207 w209] -> w199
      frame False {
        # "Sleep for 500ms"
        n90 = property on="Camera Image" class="ImageControl"("ROI"=T17 {"Global Rectangle"=[], "Contours"=[]}) -> ()  [unwired: 2 in, 2 out]
        n91 = Wait Until Next ms Multiple(millisecond multiple=u32 500) -> ()  [unwired: 1 out]
      }
      frame True {
        # "Here is where you would annotate,\npossibly process, and display the image"
        # "Update Mbps LED"
        n92 = call "IMAQ Clear Overlay"("Image"=w210) -> ("error out"=w211:errorcluster, "Image Out"=w209:T6)  [unwired: 2 in, 7 out]
        n93 = Unbundle By Name(w211) -> ("status"=w212:bool)
        n94 = property on="Image Message" class="Str"("Visible"=w212) -> ()  [unwired: 2 in, 2 out]
      }
    }
    "Camera Image" <- w199
    n95 = call <vilib>:"WPI_DashboardFormatPerf.vi"("Right Camera Perf"=w192, "Performance"=w193, "String in"=w191) -> ()  [unwired: 9 in]
  }
  n96 = call "Handle Camera Configuration.vi"("CameraNameRef"=w8, "Display Name"=w3, "ClusterRef"=w9) -> ()  [unwired: 9 in]
  n97 = while {
    tunnel: w11 -> [w227]
    tunnel: w10 -> [_]
    tunnel: [w222] -> _
    tunnel: w4 -> [w218]
    tunnel: w3 -> [w215]
    i -> [w222]
    stop <- FALSE stop-if-true
    n98 = local read "NT Connection"() -> (w219:bool)
    n99 = local read "Rec Mode"() -> (w226:enum32{"Stop", "Record", "Playback"})
    n100 = Bundle("Camera Name Right"="Camera Name Right", w215, "Saved DB Images Info"=w218) -> (w217:T19)  [unwired: 1 in]
    n101 = call <vilib>:"WPI_CameraRead MJPG for Dashboard_2.vi"("Camera Settings"="Camera Settings Right", "Rec Mode"=w226, "NT Connection"=w219, "Capture Info"=w217, "Image in"=w227) -> ("perf info"=w213:cluster{"Bandwidth (Mbps)":dbl, "fps":dbl}, "Active"=w221:bool, "Image\\ out"=w224:T6)  [unwired: 4 in]
    n102 = case shown="False" w221 {
      tunnel: w224 -> [w229 w232]
      tunnel: [w229 w232] -> w220
      tunnel: [_ w231] -> w214
      tunnel: w213 -> [_ w231]
      frame False {
        n103 = Wait Until Next ms Multiple(millisecond multiple=u32 500) -> ()  [unwired: 1 out]
        n104 = property on="Camera Image Right" class="ImageControl"("ROI"=T17 {"Global Rectangle"=[], "Contours"=[]}) -> ()  [unwired: 2 in, 2 out]
      }
      frame True {
      }
    }
    "Camera Image Right" <- w220
    "Right Camera Perf" <- w214
  }
  n105 = register-events(refnum<vi> refnum) -> (reference out=w49:refnum<event-registration>, error out=w48:errorcluster)  [unwired: 2 in]
  n106 = call "Initialize Camera and CheckList.vi"("ListBox in"=w35) -> ()  [unwired: 11 in]
  n107 = call "Adjust Dashboard Window_NO_RESIZE.vi"("Sizing Refnums"=w36, "Size Constraints"=w38, "VI"=w45, "WIn Mode"=w23) -> ()  [unwired: 8 in]
  n108 = call <vilib>:"NT Bind Controls to SmartDashboard.vi"("Bound Control Refs"=w43) -> ()  [unwired: 11 in]
  n109 = vi-ref "Playback Controls.vi"() -> (w50:refnum<vi>)
  n110 = property class="VI"() -> ("Panel"=w52:refnum<vi>)  [unwired: 2 in, 2 out]
  n111 = call "FieldDisplaySmall.vi"() -> ()  [unwired: 1 in]
  n112 = property class="Pnl"(reference=w52) -> ("Panes[]"=w53:refnum<vi>[])  [unwired: 1 in, 2 out]
  n113 = disable-structure shown="Disabled" {
    frame Disabled {
      n114 = call "DriveModuleTrend.vi"("Module"=0) -> ()  [unwired: 11 in]
      n115 = call "DriveModuleTrend.vi"("Module"=1) -> ()  [unwired: 11 in]
      n116 = call "DriveModuleTrend.vi"("Module"=2) -> ()  [unwired: 11 in]
      n117 = call "DriveModuleTrend.vi"("Module"=3) -> ()  [unwired: 11 in]
    }
    frame Enabled {
    }
  }
  n118 = Index Array(array=w53) -> (element=w51:refnum<vi>)  [unwired: 1 in]
  n119 = control-ref of="Test Tree"() -> (w54:refnum<vi>)
  n120 = while {
    tunnel: [w242] -> _
    tunnel: w54 -> [w241]
    tunnel: w50 -> [w240]
    tunnel: w49 -> [w239]
    tunnel: w48 -> [_]
    tunnel: w45 -> [w238]
    tunnel: w1 -> [w237]
    i -> [w242]
    stop <- FALSE stop-if-true
    n121 = event shown="[0] Timeout" {
      selector: w239 -> [_ _ _ _ _ _ _ _ _ _ _ _ _ _ _ _ _]
      dyn-events: [_ _ _ _ _ _ _ _ _ _ _ _ _ w449 _ _ _] -> _
      timeout: u32 60 ("milliseconds to wait") -> [_ _ _ _ _ _ _ _ _ _ _ _ _ _ _ _ _]
      tunnel: w241 -> [w252 _ _ _ _ _ _ _ _ _ _ _ _ _ _ _ _]
      tunnel: "Test Tree" -> [_ _ _ _ _ _ _ _ w422 w429 w430 w433 w440 _ _ _ _]
      tunnel: w240 -> [_ _ _ _ _ _ _ _ _ _ _ _ _ w451 _ w466 _]
      tunnel: w238 -> [_ _ _ _ _ _ _ _ _ _ _ _ _ w447 _ _ _]
      tunnel: w237 -> [w247 _ _ _ _ _ _ _ _ _ _ _ _ _ _ _ _]
      event Timeout {
        n122 = event-data() -> ()  [unwired: 1 in, 1 out]
        n123 = local read "Mode"() -> (w250:T5)
        n124 = case shown="\"Variables\"" "Dashboard Tab" {
          tunnel: w252 -> [_ _ w269 _]
          tunnel: "/TestMode/Automatic/" ("Name Pattern") -> [_ _ w268 _]
          tunnel: T20 [{"Operation"=enum."Clear", "Color Box"=14013909}, {"Operation"=enum."Clear", "Color Box"=14013909}, {"Operation"=enum."Clear", "Color Box"=14013909}, {"Operation"=enum."Clear", "Color Box"=14013909}, {"Operation"=enum."Update", "Color Box"=14013909}, {"Operation"=enum."Update", "Color Box"=16777215}, {"Operation"=enum."Clear", "Color Box"=14013909}, {"Operation"=enum."Clear", "Color Box"=14013909}, {"Operation"=enum."Clear", "Color Box"=14013909}] -> [_ _ w261 _]
          tunnel: w250 -> [_ _ w260 _]
          tunnel: u32[] [15790320, 15790320, 15790320, 15790320, 16777215, 16777215, 15790320, 15790320, 15790320] -> [_ _ _ _]
          tunnel: w247 -> [_ w254 _ _]
          frame "Custom", Default {
          }
          frame "Basic" {
            n125 = disable-structure shown="Disabled" {
              disable-tunnel: w254 -> [w255 _]
              frame Disabled {
                n126 = call <vilib>:"WPI_DashboardUpdateNames.vi"("Controls on Tab"=w255) -> ()  [unwired: 11 in]
              }
              frame Enabled {
              }
            }
          }
          frame "Test" {
            w267 = -2 ("Active Item:Row Number")
            n127 = Index Array(array=w261, index=w260) -> (element=w262:T23)
            n128 = Unbundle(w262) -> ("Operation"=w263:enum16{"Update", "Clear"}, "Color Box"=w264:u32)
            n129 = call <vilib>:"NT Read String.vi"("name"="TestMode/TestName" ("Name")) -> ("value"=w258:string)  [unwired: 8 in, 2 out]
            n130 = call <vilib>:"NT Read and Format Entries as Tree.vi"("Operation"=w263, "Name Pattern"=w268, "Tree Refnum"=w269) -> ()  [unwired: 7 in, 2 out]
            n131 = case shown="\"\"" w258 {
              tunnel: "TestMode/TestProgress" ("Name") -> [w271 _]
              tunnel: "TestMode/TestProgressText" ("Name") -> [w270 _]
              frame Default {
                n132 = call <vilib>:"NT Read Number.vi"("name"=w271) -> ("value"=w272:dbl)  [unwired: 8 in, 2 out]
                n133 = call <vilib>:"NT Read String.vi"("name"=w270) -> ("value"=w273:string)  [unwired: 8 in, 2 out]
                n134 = Bundle("value"=w272, "value"=w273) -> (→"Progress":cluster{"value":dbl, "value":string})  [unwired: 1 in]
              }
              frame "" {
                n135 = property on="Progress" class="Clust (strict)"("Visible"=FALSE) -> ()  [unwired: 2 in, 2 out]
                n136 = local write "Test Name"(u16 0) -> ()
              }
            }
            n137 = property on="Test Tree" class="Tree (strict)"("Active Item Row Number"=w267, "ActiveColNum"=w267, "CellBG"=w264, "Active Item Row Number"=-1 ("Active Item:Row Number"), "CellBG"=u32 5789784 ("Color Box")) -> ()  [unwired: 2 in, 2 out]
          }
          frame "Variables" {
            w278 = string[] ["CameraPublisher", "Usage", "DB", "schema", "cameraPublisher", "photonvision"]  # Items to initially close
            # "#NOTE JAS for now..."
            n138 = control-ref of="Tree"() -> (w282:refnum<vi>)
            n139 = First Call?() -> (First Call?: T/F=w281:bool)
            n140 = Select(t=w278, s=w281, f=string[] []) -> (s? t:f=w280:string[])
            n141 = call <vilib>:"NT Read and Format Entries as Tree.vi"("Tags to  Close"=w280, "Name Pattern"="/SmartDashboard/", "Tree Refnum"=w282) -> ()  [unwired: 7 in, 2 out]
          }
        }
        n142 = call <vilib>:"NT Connection Info.vi"() -> ("Connected"=→"NT Connection":bool)  [unwired: 11 in]
      }
      event "Test Tree": Value Change {
        # "Show appropriate\ncontrols"
        n143 = event-data() -> ("CtlRef"=w286:refnum<vi>, "NewVal"=w284:string)  [unwired: 1 in]
        n144 = call <vilib>:"WPI_UtilitiesGetTreeIOName.vi"("NewVal"=w284, "TreeControl in"=w286) -> ("I/O Name"=w287:string)  [unwired: 9 in]
        n145 = case shown="\"Camera\"" w287 {
          selector: w287 -> [_ w294 _ w316 w325 _]
          tunnel: w284 -> [_ _ w313 w315 _ w332]
          tunnel: cluster{string[]}[] [{["640x480", "320x240", "160x120"]}, {["Auto", "Fixed indoor", "Fixed outdoor 1", "Fixed outdoor 2", "Fixed fluorescent 1", "Fixed fluorescent 2", "Hold current"]}, {["Auto", "Flicker-free 50 Hz", "Flicker-free 60 Hz", "Hold current"]}, {["None", "Prioritize frame rate", "Prioritize image quality"]}, {["Monochrome", "Color"]}] -> [_ _ _ _ _ w331]
          frame Default {
            w289 = FALSE ("Visible")
            w288 = FALSE ("Visible")
            n146 = property on="Motor" class="Clust (strict)"("Visible"=w288) -> ()  [unwired: 2 in, 2 out]
            n147 = property on="Test Ring" class="Ring (strict)"("Visible"=w288) -> ()  [unwired: 2 in, 2 out]
            n148 = property on="Rev/Fwd" class="Clust (strict)"("Visible"=w289) -> ()  [unwired: 2 in, 2 out]
            n149 = property on="On/Off" class="Bool (strict)"("Visible"=w289) -> ()  [unwired: 2 in, 2 out]
            n150 = property on="Test Slider" class="Slide (strict)"("Visible"=w289) -> ()  [unwired: 2 in, 2 out]
          }
          frame "Analog Out", "Motor", "PWM" {
            w295 = FALSE ("Visible")
            n151 = case shown="\"Analog Out\"" w294 {
              tunnel: [1.0 ("Value") -1.0 ("Value") 0.0 ("Value")] -> w293
              tunnel: [255.0 ("Value") 1.0 ("Value") 5.0 ("Value")] -> w292
              tunnel: [128.0 ("Value") 0.0 ("Value") 0.0 ("Value")] -> w291
              tunnel: [64.0 ("Value") 0.5 ("Value") 1.0 ("Value")] -> w290
              frame "PWM" {
              }
              frame "Motor", Default {
              }
              frame "Analog Out" {
              }
            }
            n152 = property on="Motor" class="Clust (strict)"("Visible"=TRUE) -> ()  [unwired: 2 in, 2 out]
            n153 = property on="Value" class="Slide (strict)"("Value"=w291, "Scale.Minimum"=w293, "Scale.Maximum"=w292, "Scale.Increment"=w290) -> ()  [unwired: 2 in, 2 out]
            n154 = property on="On/Off" class="Bool (strict)"("Visible"=w295) -> ()  [unwired: 2 in, 2 out]
            n155 = property on="Test Slider" class="Slide (strict)"("Visible"=w295) -> ()  [unwired: 2 in, 2 out]
            n156 = property on="Test Ring" class="Ring (strict)"("Visible"=w295) -> ()  [unwired: 2 in, 2 out]
            n157 = property on="Rev/Fwd" class="Clust (strict)"("Visible"=w295) -> ()  [unwired: 2 in, 2 out]
          }
          frame "Servo" {
            w311 = FALSE ("Visible")
            n158 = call <vilib>:"NT Read Number.vi"("name"=w313) -> ("value"=w312:dbl)  [unwired: 8 in, 2 out]
            n159 = property on="Test Slider" class="Slide (strict)"("Visible"=TRUE, "Scale.Maximum"=170.0 ("Scale.Range:Maximum")) -> ()  [unwired: 2 in, 2 out]
            n160 = local write "Test Slider"(w312) -> ()
            n161 = property on="Motor" class="Clust (strict)"("Visible"=w311) -> ()  [unwired: 2 in, 2 out]
            n162 = property on="Rev/Fwd" class="Clust (strict)"("Visible"=w311) -> ()  [unwired: 2 in, 2 out]
            n163 = property on="On/Off" class="Bool (strict)"("Visible"=w311) -> ()  [unwired: 2 in, 2 out]
            n164 = property on="Test Ring" class="Ring (strict)"("Visible"=w311) -> ()  [unwired: 2 in, 2 out]
          }
          frame "Relay", "Solenoid" {
            w314 = FALSE ("Visible")
            n165 = property on="Motor" class="Clust (strict)"("Visible"=w314) -> ()  [unwired: 2 in, 2 out]
            n166 = property on="Test Slider" class="Slide (strict)"("Visible"=w314) -> ()  [unwired: 2 in, 2 out]
            n167 = Search and Replace String(input string=w315, search string="/Value  **", replace string="/Direction") -> (result string=w321:string)  [unwired: 5 in, 3 out]
            n168 = property on="Test Ring" class="Ring (strict)"("Visible"=w314) -> ()  [unwired: 2 in, 2 out]
            n169 = call <vilib>:"NT Read String.vi"("name"=w321) -> ("value"=w319:string)  [unwired: 8 in, 2 out]
            n170 = Equal?(x="Both directions", y=w319) -> (x = y?=w317:bool)
            n171 = Not(x=w317) -> (.not. x?=w318:bool)
            n172 = property on="Rev/Fwd" class="Clust (strict)"("Visible"=w317) -> ()  [unwired: 2 in, 2 out]
            n173 = property on="On/Off" class="Bool (strict)"("Visible"=w318, "Caption.Text"=w316) -> ()  [unwired: 2 in, 2 out]
          }
          frame "Compressor", "Digital Out" {
            w324 = FALSE ("Visible")
            # "Get direction and finish"
            n174 = property on="Motor" class="Clust (strict)"("Visible"=w324) -> ()  [unwired: 2 in, 2 out]
            n175 = property on="Test Slider" class="Slide (strict)"("Visible"=w324) -> ()  [unwired: 2 in, 2 out]
            n176 = property on="Test Ring" class="Ring (strict)"("Visible"=w324) -> ()  [unwired: 2 in, 2 out]
            n177 = property on="On/Off" class="Bool (strict)"("Visible"=TRUE, "Caption.Text"=w325) -> ()  [unwired: 2 in, 2 out]
            n178 = property on="Rev/Fwd" class="Clust (strict)"("Visible"=FALSE) -> ()  [unwired: 2 in, 2 out]
          }
          frame "Camera" {
            n179 = call <vilib>:"NT_Get Last Path Segment.vi"("String in"=w332) -> ("String out"=w333:string)  [unwired: 10 in]
            n180 = property on="On/Off" class="Bool (strict)"("Visible"=FALSE) -> ()  [unwired: 2 in, 2 out]
            n181 = property on="Motor" class="Clust (strict)"("Visible"=FALSE) -> ()  [unwired: 2 in, 2 out]
            n182 = property on="Rev/Fwd" class="Clust (strict)"("Visible"=FALSE) -> ()  [unwired: 2 in, 2 out]
            n183 = case shown="\"White Balance  **\"" w333 {
              tunnel: w332 -> [w339 w348 w357 w366 w375 _ w381]
              tunnel: w331 -> [w337 w345 w354 w363 w372 _ _]
              frame "Size  **" {
                n184 = Index Array(array=w337) -> (element=w336:cluster{string[]})  [unwired: 1 in]
                n185 = call <vilib>:"NT Read String.vi"("name"=w339) -> ("value"=w338:string)  [unwired: 8 in, 2 out]
                n186 = Unbundle(w336) -> (w334:string[])
                n187 = Match First String(2:w334, 3:w338) -> (0:w335:i32)  [unwired: 1 out]
                n188 = property on="Test Ring" class="Ring (strict)"("Value"=w335, "Strings []"=w334) -> ()  [unwired: 2 in, 2 out]
                n189 = property on="Test Ring" class="Ring (strict)"("Visible"=TRUE) -> ()  [unwired: 2 in, 2 out]
                n190 = property on="Test Slider" class="Slide (strict)"("Visible"=FALSE) -> ()  [unwired: 2 in, 2 out]
              }
              frame "White Balance  **" {
                n191 = Index Array(array=w345, index=1) -> (element=w346:cluster{string[]})
                n192 = call <vilib>:"NT Read String.vi"("name"=w348) -> ("value"=w347:string)  [unwired: 8 in, 2 out]
                n193 = Unbundle(w346) -> (w343:string[])
                n194 = Match First String(2:w343, 3:w347) -> (0:w342:i32)  [unwired: 1 out]
                n195 = property on="Test Ring" class="Ring (strict)"("Value"=w342, "Strings []"=w343) -> ()  [unwired: 2 in, 2 out]
                n196 = property on="Test Ring" class="Ring (strict)"("Visible"=TRUE) -> ()  [unwired: 2 in, 2 out]
                n197 = property on="Test Slider" class="Slide (strict)"("Visible"=FALSE) -> ()  [unwired: 2 in, 2 out]
              }
              frame "Exposure  **" {
                n198 = Index Array(array=w354, index=2) -> (element=w355:cluster{string[]})
                n199 = call <vilib>:"NT Read String.vi"("name"=w357) -> ("value"=w356:string)  [unwired: 8 in, 2 out]
                n200 = Unbundle(w355) -> (w351:string[])
                n201 = Match First String(2:w351, 3:w356) -> (0:w352:i32)  [unwired: 1 out]
                n202 = property on="Test Ring" class="Ring (strict)"("Value"=w352, "Strings []"=w351) -> ()  [unwired: 2 in, 2 out]
                n203 = property on="Test Ring" class="Ring (strict)"("Visible"=TRUE) -> ()  [unwired: 2 in, 2 out]
                n204 = property on="Test Slider" class="Slide (strict)"("Visible"=FALSE) -> ()  [unwired: 2 in, 2 out]
              }
              frame "Exposure Priority  **" {
                n205 = Index Array(array=w363, index=3) -> (element=w364:cluster{string[]})
                n206 = call <vilib>:"NT Read String.vi"("name"=w366) -> ("value"=w365:string)  [unwired: 8 in, 2 out]
                n207 = Unbundle(w364) -> (w360:string[])
                n208 = Match First String(2:w360, 3:w365) -> (0:w361:i32)  [unwired: 1 out]
                n209 = property on="Test Ring" class="Ring (strict)"("Value"=w361, "Strings []"=w360) -> ()  [unwired: 2 in, 2 out]
                n210 = property on="Test Ring" class="Ring (strict)"("Visible"=TRUE) -> ()  [unwired: 2 in, 2 out]
                n211 = property on="Test Slider" class="Slide (strict)"("Visible"=FALSE) -> ()  [unwired: 2 in, 2 out]
              }
              frame "Color Enable  **" {
                n212 = Index Array(array=w372, index=4) -> (element=w373:cluster{string[]})
                n213 = call <vilib>:"NT Read String.vi"("name"=w375) -> ("value"=w374:string)  [unwired: 8 in, 2 out]
                n214 = Unbundle(w373) -> (w369:string[])
                n215 = Match First String(2:w369, 3:w374) -> (0:w370:i32)  [unwired: 1 out]
                n216 = property on="Test Ring" class="Ring (strict)"("Value"=w370, "Strings []"=w369) -> ()  [unwired: 2 in, 2 out]
                n217 = property on="Test Ring" class="Ring (strict)"("Visible"=TRUE) -> ()  [unwired: 2 in, 2 out]
                n218 = property on="Test Slider" class="Slide (strict)"("Visible"=FALSE) -> ()  [unwired: 2 in, 2 out]
              }
              frame Default {
                n219 = property on="Test Ring" class="Ring (strict)"("Visible"=FALSE) -> ()  [unwired: 2 in, 2 out]
                n220 = property on="Test Slider" class="Slide (strict)"("Visible"=FALSE) -> ()  [unwired: 2 in, 2 out]
              }
              frame "Brightness  **", "Color Level  **", "Compression  **", "FPS  **", "Sharpness  **" {
                n221 = call <vilib>:"NT Read Number.vi"("name"=w381) -> ("value"=w380:dbl)  [unwired: 8 in, 2 out]
                n222 = local write "Test Slider"(w380) -> ()
                n223 = property on="Test Ring" class="Ring (strict)"("Visible"=FALSE) -> ()  [unwired: 2 in, 2 out]
                n224 = property on="Test Slider" class="Slide (strict)"("Visible"=TRUE, "Scale.Maximum"=100.0 ("Scale.Range:Maximum")) -> ()  [unwired: 2 in, 2 out]
              }
            }
          }
        }
        n225 = property on="Progress" class="Clust (strict)"("Visible"=FALSE) -> ()  [unwired: 2 in, 2 out]
      }
      event "Test Name": Mouse Enter {
        # "Populate the ring with the list of tests"
        n226 = event-data() -> ()  [unwired: 1 in, 1 out]
        n227 = call <vilib>:"NT Read String Array.vi"("name"="TestMode/TestList" ("Name")) -> ("value"=w388:string[])  [unwired: 8 in, 2 out]
        n228 = Build Array (concatenate)("Select the test to run...", w388) -> (w387:string[])
        n229 = property on="Test Name" class="Ring (strict)"("Strings []"=w387) -> ()  [unwired: 2 in, 2 out]
      }
      event "Test Name": Value Change {
        w389 = FALSE ("Visible")
        # "Tell the robot the test name to run"
        n230 = event-data() -> ("NewVal"=w393:u16)  [unwired: 1 in]
        n231 = property on="Test Name" class="Ring (strict)"() -> ("Strings []"=w394:string[])  [unwired: 2 in, 2 out]
        n232 = local write "Progress"(T8 {"Test Progress"=0, "Test Progress Text"=""} ("Progress")) -> ()
        n233 = Index Array(array=w394, index=w393) -> (element=w392:string)
        n234 = call <vilib>:"NT Write String.vi"("value"=w392, "name"="TestMode/TestName" ("Name")) -> ()  [unwired: 9 in, 1 out]
        n235 = property on="Progress" class="Clust (strict)"("Visible"=TRUE) -> ()  [unwired: 2 in, 2 out]
        n236 = property on="Motor" class="Clust (strict)"("Visible"=w389) -> ()  [unwired: 2 in, 2 out]
        n237 = property on="Test Slider" class="Slide (strict)"("Visible"=w389) -> ()  [unwired: 2 in, 2 out]
        n238 = property on="On/Off" class="Bool (strict)"("Visible"=w389) -> ()  [unwired: 2 in, 2 out]
        n239 = property on="Rev/Fwd" class="Clust (strict)"("Visible"=w389) -> ()  [unwired: 2 in, 2 out]
        n240 = property on="Test Ring" class="Ring (strict)"("Visible"=w389) -> ()  [unwired: 2 in, 2 out]
      }
      event "Select Auto": Mouse Enter {
        # "Populate the combo box with the list of autonomous options"
        n241 = event-data() -> ()  [unwired: 1 in, 1 out]
        n242 = call <vilib>:"NT Read String Array.vi"("name"="Auto List" ("Name")) -> ("value"=w396:string[])  [unwired: 8 in, 2 out]
        n243 = property on="Select Auto" class="CmbBox"("Strings[]"=w396) -> ()  [unwired: 2 in, 2 out]
      }
      event "Select Auto": Value Change {
        # "User modified the Auto Selection. Write to NT variable so robot knows."
        n244 = event-data() -> ("NewVal"=w398:string)  [unwired: 1 in]
        n245 = call <vilib>:"NT Write String.vi"("value"=w398, "name"="Auto Selector" ("Name")) -> ()  [unwired: 9 in, 1 out]
      }
      event "CheckList": Double Click {
        # "Shift clears all"
        # "Update symbols on the listbox"
        n246 = event-data() -> ("PlatMods.Shift"=w400:bool, "Row"=w402:i32)  [unwired: 1 in]
        n247 = case shown="True" w400 {
          tunnel: w402 -> [w406 _]
          tunnel: 1 -> [w405 _]
          frame False {
            n248 = property on="CheckList" class="LstBox (strict)"() -> ("Item Symbols"=w404:i32[])  [unwired: 2 in, 2 out]
            n249 = Replace Array Subset(array=w404, new element=w405, index=w406) -> (w403:i32[])
            n250 = property on="CheckList" class="LstBox (strict)"("Item Symbols"=w403) -> ()  [unwired: 2 in, 2 out]
          }
          frame True {
            w407 = 0 ("Top Row")
            n251 = property on="CheckList" class="LstBox (strict)"() -> ("Number of Rows"=w409:u32)  [unwired: 2 in, 2 out]
            n252 = Initialize Array(0, w409) -> (w408:i32[])
            n253 = property on="CheckList" class="LstBox (strict)"("Top Row"=w407, "Value"=w407, "Item Symbols"=w408) -> ()  [unwired: 2 in, 2 out]
          }
        }
      }
      event "CheckList": Key Down {
        # "Update symbols on the listbox\nLeft and right keys check and uncheck"
        n254 = event-data() -> ("VKey"=w412:T21)  [unwired: 1 in]
        n255 = case shown="\"Left\", \"Right\"" w412 {
          selector: w412 -> [w417 _]
          tunnel: eventvkey."Left" ("VKey") -> [w415 _]
          frame "Left", "Right" {
            n256 = Equal?(x=w415, y=w417) -> (x = y?=w416:bool)
            n257 = Select(t=0, s=w416, f=1) -> (s? t:f=w418:i32)
            n258 = property on="CheckList" class="LstBox (strict)"() -> ("Item Symbols"=w421:i32[])  [unwired: 2 in, 2 out]
            n259 = Replace Array Subset(array=w421, new element=w418, index="CheckList") -> (w420:i32[])
            n260 = property on="CheckList" class="LstBox (strict)"("Item Symbols"=w420) -> ()  [unwired: 2 in, 2 out]
          }
          frame Default {
          }
        }
      }
      event "Motor.Enable": Value Change {
        # "When the test mode otor enable helper is set, update that\ntree row item's value"
        n261 = event-data() -> ("NewVal"=w426:bool)  [unwired: 1 in]
        n262 = Unbundle("Motor") -> ("Value"=w425:dbl)  [unwired: 1 out]
        n263 = Select(t=w425, s=w426, f=0.0) -> (s? t:f=w423:dbl)
        n264 = call <vilib>:"NT Write Number.vi"("value"=w423, "name"=w422) -> ()  [unwired: 9 in, 1 out]
      }
      event "Test Slider": Value Change {
        # "When the test mode slider helper is set, update that\ntree row item's value"
        n265 = event-data() -> ("NewVal"=w428:dbl)  [unwired: 1 in]
        n266 = call <vilib>:"NT Write Number.vi"("value"=w428, "name"=w429) -> ()  [unwired: 9 in, 1 out]
      }
      event "On/Off": Value Change {
        # "When the test mode on/off helper value is set, update that\ntree row item's value"
        n267 = event-data() -> ("NewVal"=w432:bool)  [unwired: 1 in]
        n268 = Boolean To (0,1)(Boolean=w432) -> (0, 1=w431:i16)
        n269 = call <vilib>:"NT Write Number.vi"("value"=w431, "name"=w430) -> ()  [unwired: 9 in, 1 out]
      }
      event "Rev/Fwd": Value Change {
        # "When the test mode helper value for relays is set, update that\ntree row item's value"
        n270 = event-data() -> ("NewVal.Forward"=w439:bool, "NewVal.Reverse"=w438:bool)  [unwired: 1 in]
        n271 = Boolean To (0,1)(Boolean=w439) -> (0, 1=w435:i16)
        n272 = Boolean To (0,1)(Boolean=w438) -> (0, 1=w437:i16)
        n273 = Negate(x=w437) -> (-x=w436:i16)
        n274 = Add(x=w435, y=w436) -> (x+y=w434:i16)
        n275 = call <vilib>:"NT Write Number.vi"("value"=w434, "name"=w433) -> ()  [unwired: 9 in, 1 out]
      }
      event "Test Ring": Value Change {
        # "When a test mode helper value is selected from the ring,\nset the tree item's variable to the string value"
        n276 = event-data() -> ("NewVal"=w442:u16)  [unwired: 1 in]
        n277 = property on="Test Ring" class="Ring (strict)"() -> ("Strings []"=w443:string[])  [unwired: 2 in, 2 out]
        n278 = Index Array(array=w443, index=w442) -> (element=w441:string)
        n279 = call <vilib>:"NT Write String.vi"("value"=w441, "name"=w440) -> ()  [unwired: 9 in, 1 out]
      }
      event "Rec Mode": Value Change {
        # "Update globals for recording mode and path to read log from.\nClear when logging and let NetworkTables set path for vision to\nuse."
        n280 = event-data() -> ("NewVal"=w452:enum32{"Stop", "Record", "Playback"})  [unwired: 1 in]
        n281 = global write "WPI_DashboardLogging Global.vi" "Logging Filename"(path "") -> ()
        n282 = global write "WPI_DashboardLogging Global.vi" "Recording"(w452) -> ()
        n283 = case shown="\"Playback\"" w452 {
          tunnel: w451 -> [_ w454 w462]
          tunnel: [_ _ w461] -> w449
          tunnel: [_ _ w460] -> _
          tunnel: w447 -> [_ _ w458]
          tunnel: cluster{i32, i32} {-250, 170} -> [_ _ w457]
          tunnel: [_ _ T22 {"Image Size"=TRUE, "Image Type"=TRUE, "Pixel Value"=TRUE, "ROI Information"=TRUE, "Zoom Factor"=FALSE} ("Image Information Shown:All Elements")] -> w444
          tunnel: [_ _ TRUE ("Zoom Factor")] -> w445
          frame Default {
          }
          frame "Stop", "Record" {
            # "Place Window too"
            n284 = invoke class="VI" method="FP.Close"(reference=w454) -> (reference out=w453:refnum<vi>)  [unwired: 2 in, 2 out]
            n285 = invoke class="VI" method="Abort VI"(reference=w453) -> ()  [unwired: 2 in, 3 out]
          }
          frame "Playback" {
            n286 = call "Open Playback Panel.vi"("Offset"=w457, "DB VI Ref"=w458, "Playback in"=w462) -> ("Playback out"=w459:refnum<vi>)  [unwired: 8 in]
            n287 = register-events(w459) -> (reference out=w461:refnum<event-registration>, error out=w460:errorcluster)  [unwired: 2 in]
          }
        }
        n288 = property on="Camera Image Right" class="ImageControl"("Image Information Shown"=w444, "Image Information Visible"=w445) -> ()  [unwired: 2 in, 2 out]
        n289 = property on="Camera Image" class="ImageControl"("Image Information Shown"=w444, "Image Information Visible"=w445) -> ()  [unwired: 2 in, 2 out]
        n290 = call <vilib>:"WPI_DashboardNT Log FieldName Cache.vi"("Operation"=enum16{"Lookup/Add", "Index", "Clear"}."Clear") -> ()  [unwired: 8 in, 3 out]
      }
      event Panel Close {
        w463 = enum32{"Stop", "Record", "Playback"}."Stop" ("Rec Mode")
        # "Playback window has been closed, abort"
        n291 = event-data() -> ()  [unwired: 1 in, 4 out]
        n292 = local write "Rec Mode"(w463) -> ()
        n293 = global write "WPI_DashboardLogging Global.vi" "Recording"(w463) -> ()
      }
      event Panel Close {
        # "Abort playback window and ourself"
        n294 = event-data() -> ()  [unwired: 1 in, 4 out]
        n295 = invoke class="VI" method="FP.Close"(reference=w466) -> (reference out=w465:refnum<vi>)  [unwired: 2 in, 2 out]
        n296 = invoke class="VI" method="Abort VI"(reference=w465) -> (error out=w464:errorcluster)  [unwired: 2 in, 2 out]
        n297 = invoke class="VI" method="Abort VI"(error in=w464) -> ()  [unwired: 2 in, 3 out]
      }
      event "Tree": Double Click {
        n298 = event-data() -> ("PlatMods"=w472:T24, "Tag"=w469:string)  [unwired: 1 in]
        n299 = Unbundle(w472) -> ("Shift"=w471:bool)  [unwired: 4 out]
        n300 = String Subset(string=w469, length (rest)=1 ("length (rest)")) -> (substring=w468:string)  [unwired: 1 in]
        n301 = Not(x=w471) -> (.not. x?=w470:bool)
        n302 = case shown="\"/\"" w468 {
          tunnel: w469 -> [_ w474]
          tunnel: w470 -> [_ w473]
          frame Default {
          }
          frame "/" {
            n303 = call <vilib>:"NT Update Persistence.vi"("Persistence"=w473, "Name"=w474) -> ()  [unwired: 9 in, 1 out]
          }
        }
      }
    }
  }
  n304 = while {
    tunnel: w51 -> [w476]
    i -> [w479]
    stop <- FALSE stop-if-true
    n305 = Wait (ms)(milliseconds to wait=u32 100) -> ()  [unwired: 1 out]
    n306 = case shown="\"Playback\"" "Rec Mode" {
      tunnel: w479 -> [_ _ w494]
      tunnel: [u32 2829099 ("Base Color") u32 11141120 ("Target Color") w483] -> w475
      frame "Stop", Default {
        # "Reset the color, extra updates don't cost much"
      }
      frame "Record" {
      }
      frame "Playback" {
        # "Playback"
        n307 = Quotient & Remainder(x=w494, y=u32 50 ("milliseconds to wait")) -> (x-y*floor(x/y)=w490:u32)  [unwired: 1 out]
        n308 = Divide(x=w490, y=u32 50 ("milliseconds to wait")) -> (x/y=w487:dbl)
        n309 = Multiply(x=6.283185307179586, y=w487) -> (x*y=w492:dbl)
        n310 = Sine(x=w492) -> (sin(x)=w491:dbl)
        n311 = Absolute Value(x=w491) -> (abs(x)=w484:dbl)
        n312 = call "Interpolate RGB Color.vi"("Proportion"=w484, "Target Color"=u32 30976, "Base Color"=u32 2829099) -> ("Result Color"=w483:u32)  [unwired: 8 in]
      }
    }
    n313 = property class="Pane"(reference=w476, "PaneColor"=w475) -> ()  [unwired: 1 in, 2 out]
  }
  n314 = local write "Dashboard Tab"(T2."Drive" ("Dashboard Tab")) -> ()
  n315 = call "TrajectoryTrend.vi"() -> ()  [unwired: 12 in]
  n316 = property on="On/Off" class="Bool (strict)"("Visible"=w24) -> ()  [unwired: 2 in, 2 out]
  n317 = property on="Motor" class="Clust (strict)"("Visible"=w24) -> ()  [unwired: 2 in, 2 out]
  n318 = property on="Progress" class="Clust (strict)"("Visible"=w24) -> ()  [unwired: 2 in, 2 out]
  n319 = property on="Test Ring" class="Ring (strict)"("Visible"=w24) -> ()  [unwired: 2 in, 2 out]
  n320 = property on="Rev/Fwd" class="Clust (strict)"("Visible"=w24) -> ()  [unwired: 2 in, 2 out]
  n321 = while {
    tunnel: u16 1741 ("timeout ms (25000)") -> [w496]
    stop <- FALSE stop-if-true
    n322 = TCP Create Listener(10:w496) -> (0:w495:errorcluster, 3:w497:refnum<k5>)  [unwired: 4 in, 1 out]
    n323 = case shown="No Error" w495 {
      selector: w495 -> [w499 _]
      tunnel: w497 -> [w500 _]
      frame No Error {
        n324 = while {
          tunnel: w500 -> [w503]
          tunnel: w499 -> [w502]
          stop <- FALSE stop-if-true
          n325 = TCP Wait On Listener(8:w502, 11:w503) -> (0:w504:errorcluster, 4:w505:refnum<k5>)  [unwired: 2 in, 3 out]
          n326 = local write "TCP"(w505) -> ()
          n327 = case shown="Error" w504 {
            frame No Error {
            }
            frame Error {
              n328 = Wait (ms)(milliseconds to wait=u32 1000) -> ()  [unwired: 1 out]
            }
          }
        }
      }
      frame Error {
        n329 = Wait (ms)(milliseconds to wait=u32 1000) -> ()  [unwired: 1 out]
      }
    }
  }
  n330 = global write "WPI_DashboardLogging Global.vi" "Recording"(w46) -> ()
  n331 = local write "Rec Mode"(w46) -> ()
  n332 = call <vilib>:"NT Write String.vi"("value"="Select Auto", "name"="Auto Selector" ("Name")) -> ()  [unwired: 9 in, 1 out]
